vi "rpm and voltage calculate from erpm.vi"(11 "E RPM":dbl) -> (1 "combustion_rpm":dbl, 2 "greater_than_0?":bool, 3 "voltage":dbl)   [LabVIEW 2014]
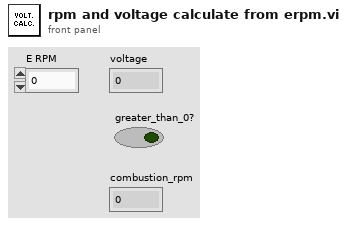
[diagram p1: front panel]
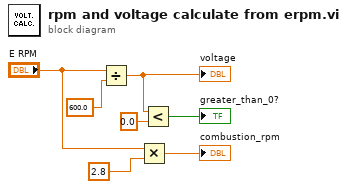
[diagram p0: block diagram]
diagram:
  n1 = Divide(x="E RPM", y=600.0) -> (x/y=w6:dbl)
  "voltage" <- w6
  n2 = Multiply(x="E RPM", y=2.8) -> (x*y=→"combustion_rpm":dbl)
  n3 = Less?(x=w6, y=0.0) -> (x < y?=→"greater_than_0?":bool)
